vi "IDE Options UI.vi"() -> ()   [LabVIEW 2020, in "Negentropic IDE.lvlib"]
uses:
  Negentropic IDE.lvlib
panel:
  in  "Override Template - Skip Open":bool
  in  "Override Template - Save Automatically":bool
  in  "Override Template - Cleaner Block Diagram":bool
  in  "Member Template - No Error Case Structure":bool
  in  "Disable All":bool
  in  "OK":bool
  # "These options can be changed from\nTools -> IlluminatedG -> IDE Options"
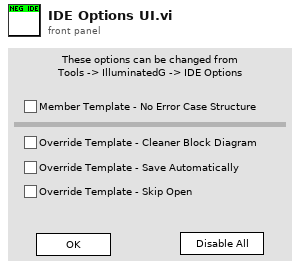
[diagram p1: front panel]
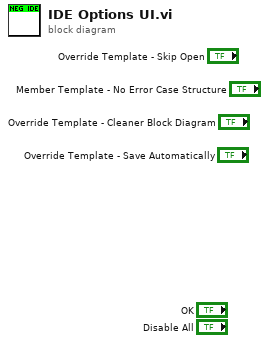
[diagram p0: block diagram]
diagram:
